vi "Top Level.vi"() -> ()   [LabVIEW 2020]
uses:
  Message.ctl
panel:
  in  "Reset DMM":bool
  out "Data":dbl
  in  "Close DMM":bool
  in  "Read DMM":bool
  in  "Init DMM":bool
  in  "Stop Button":bool
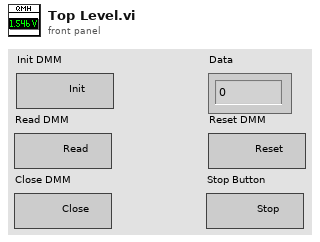
[diagram p1: front panel]
types:
  T1 = cluster{"NI":cluster{"Resource":refnum<k15>}, "Agilent":cluster{"Resource":refnum<visa-resource-name>}, "Data":dbl, "Data*":refnum<vi>, "DMM Type":string}
  T2 = typedef "Message.ctl" = cluster{"State":string, "Data":variant}
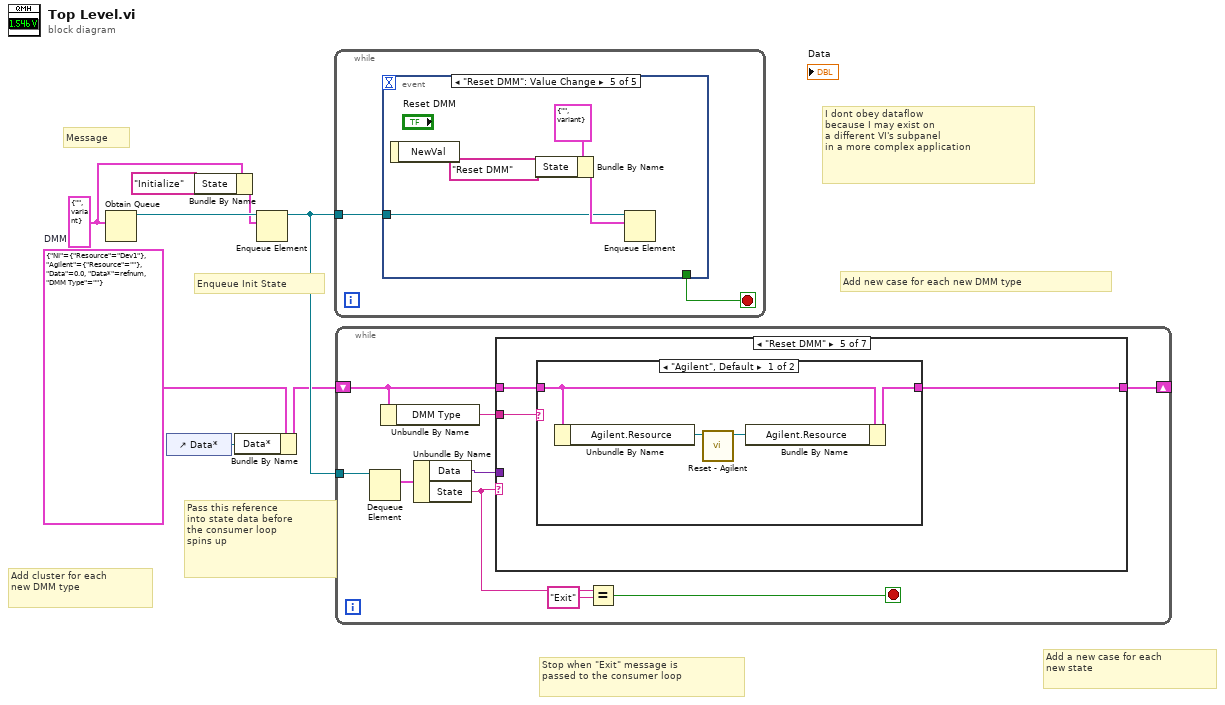
[diagram p0: block diagram]
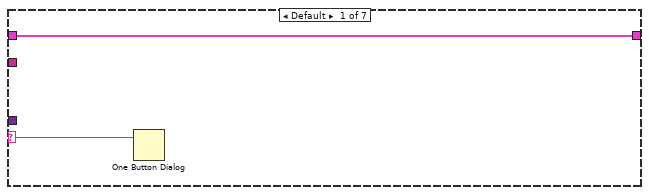
[diagram p2: hidden frame]
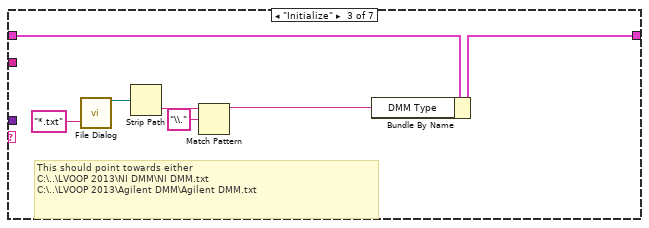
[diagram p4: hidden frame]
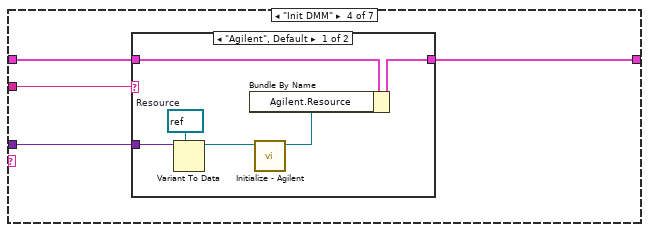
[diagram p5: hidden frame]
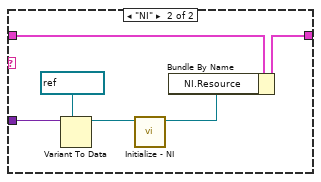
[diagram p6: hidden frame]
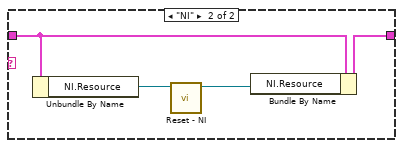
[diagram p7: hidden frame]
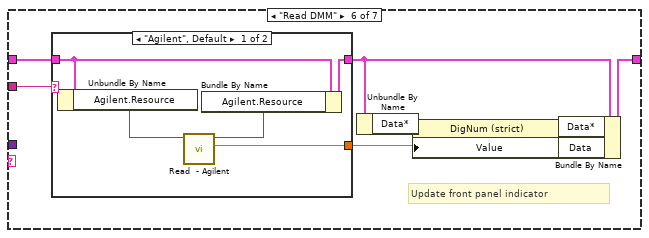
[diagram p8: hidden frame]
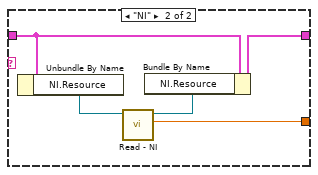
[diagram p9: hidden frame]
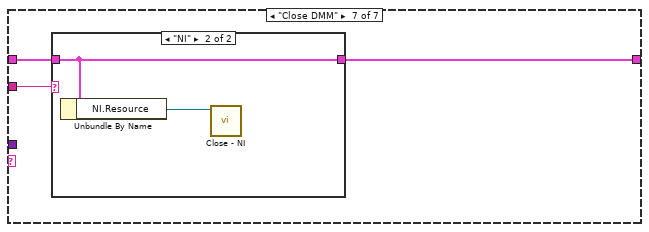
[diagram p10: hidden frame]
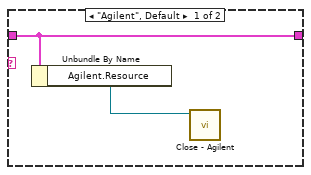
[diagram p11: hidden frame]
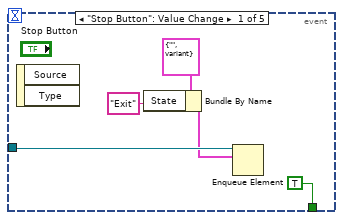
[diagram p12: hidden frame]
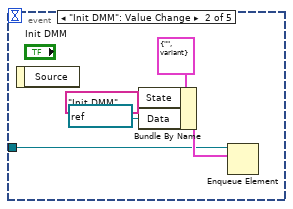
[diagram p13: hidden frame]
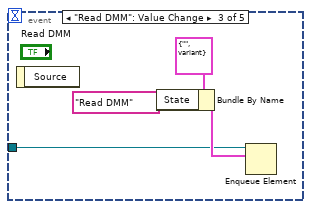
[diagram p14: hidden frame]
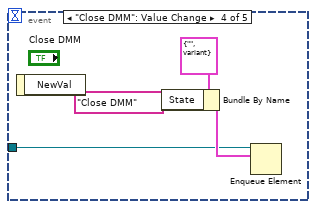
[diagram p15: hidden frame]
diagram:
  w3 = T1 {"NI"={"Resource"="Dev1"}, "Agilent"={"Resource"=""}, "Data"=0.0, "Data*"=refnum, "DMM Type"=""}  # DMM
  w6 = T2 {"State"="", "Data"=variant}
  # "I dont obey dataflow\nbecause I may exist on\na different VI's subpanel\nin a more complex application"
  # "Stop when \"Exit\" message is\npassed to the consumer loop"
  # "Add a new case for each\nnew state"
  # "Pass this reference\ninto state data before\nthe consumer loop\nspins up"
  # "Enqueue Init State"
  # "Add cluster for each\nnew DMM type"
  # "Add new case for each new DMM type"
  # "Message"
  n1 = Obtain Queue(element data type=w6) -> (queue out=w8:refnum<queue>)  [unwired: 4 in, 2 out]
  n2 = control-ref of="Data*"() -> (w1:refnum<vi>)
  n3 = Bundle By Name(cluster=w6, "State"="Initialize") -> (w5:T2)
  n4 = Bundle By Name(cluster=w3, "Data*"=w1) -> (w2:T1)
  n5 = Enqueue Element(queue=w8, element=w5) -> (queue out=w7:refnum<queue>)  [unwired: 2 in, 2 out]
  n6 = while {
    tunnel: w7 -> [w10]
    stop <- w9 stop-if-true
    n7 = event shown="[4] \"Reset DMM\": Value Change" {
      selector: _ -> [_ _ _ _ _]
      dyn-events: _ -> [_ _ _ _ _]
      timeout: _ -> [_ _ _ _ _]
      tunnel: w10 -> [w14 w17 w21 w25 w29]
      tunnel: [TRUE _ _ _ _] -> w9
      event "Stop Button": Value Change {
        n8 = event-data() -> ()  [unwired: 1 in, 2 out]
        n9 = Bundle By Name(cluster=T2 {"State"="", "Data"=variant}, "State"="Exit") -> (w12:T2)
        n10 = Enqueue Element(queue=w14, element=w12) -> ()  [unwired: 2 in, 3 out]
      }
      event "Init DMM": Value Change {
        n11 = event-data() -> ()  [unwired: 1 in, 1 out]
        n12 = Bundle By Name(cluster=T2 {"State"="", "Data"=variant}, "State"="Init DMM", "Data"=refnum<k15> "Dev1" ("Instrument Descriptor")) -> (w19:T2)
        n13 = Enqueue Element(queue=w17, element=w19) -> ()  [unwired: 2 in, 3 out]
      }
      event "Read DMM": Value Change {
        n14 = event-data() -> ()  [unwired: 1 in, 1 out]
        n15 = Bundle By Name(cluster=T2 {"State"="", "Data"=variant}, "State"="Read DMM") -> (w23:T2)
        n16 = Enqueue Element(queue=w21, element=w23) -> ()  [unwired: 2 in, 3 out]
      }
      event "Close DMM": Value Change {
        n17 = event-data() -> ()  [unwired: 1 in, 1 out]
        n18 = Bundle By Name(cluster=T2 {"State"="", "Data"=variant}, "State"="Close DMM") -> (w27:T2)
        n19 = Enqueue Element(queue=w25, element=w27) -> ()  [unwired: 2 in, 3 out]
      }
      event "Reset DMM": Value Change {
        n20 = event-data() -> ()  [unwired: 1 in, 1 out]
        n21 = Bundle By Name(cluster=T2 {"State"="", "Data"=variant}, "State"="Reset DMM") -> (w31:T2)
        n22 = Enqueue Element(queue=w29, element=w31) -> ()  [unwired: 2 in, 3 out]
      }
    }
  }
  n23 = while {
    tunnel: w7 -> [w41]
    shift-right: [w35] -> _
    shift-left: w2 -> [w34]
    stop <- w37 stop-if-true
    n24 = Dequeue Element(queue=w41) -> (element=w40:T2)  [unwired: 2 in, 3 out]
    n25 = Unbundle By Name(w34) -> ("DMM Type"=w33:string)
    n26 = Unbundle By Name(w40) -> ("Data"=w36:variant, "State"=w39:string)
    n27 = case shown="\"Reset DMM\"" w39 {
      selector: w39 -> [w43 _ _ _ _ _ _]
      tunnel: w36 -> [_ _ _ w53 _ _ _]
      tunnel: w34 -> [w42 w44 w51 w55 w70 w85 w98]
      tunnel: [w42 w44 w50 w54 w69 w83 w97] -> w35
      tunnel: w33 -> [_ _ _ w52 w68 w84 w96]
      frame Default {
        n28 = One Button Dialog(message=w43) -> ()  [unwired: 1 in, 1 out]
      }
      frame "Exit" {
      }
      frame "Initialize" {
        # "This should point towards either\nC:\\..\\LVOOP 2013\\NI DMM\\NI DMM.txt\nC:\\..\\LVOOP 2013\\Agilent DMM\\Agilent DMM.txt"
        n29 = call "File Dialog"("pattern (all files)"="*.txt") -> ("selected path"=w48:path)  [unwired: 11 in, 3 out]
        n30 = Strip Path(path=w48) -> (name=w47:string)  [unwired: 1 out]
        n31 = Match Pattern(string=w47, regular expression="\\.") -> (before substring=w45:string)  [unwired: 1 in, 3 out]
        n32 = Bundle By Name(cluster=w51, "DMM Type"=w45) -> (w50:T1)
      }
      frame "Init DMM" {
        n33 = case shown="\"Agilent\", Default" w52 {
          tunnel: w55 -> [w59 w65]
          tunnel: [w58 w64] -> w54
          tunnel: w53 -> [w60 w66]
          frame "Agilent", Default {
            w61 = refnum<visa-resource-name> refnum  # Resource
            n34 = Variant To Data(type=w61, Variant=w60) -> (data=w57:refnum<visa-resource-name>)  [unwired: 1 in, 1 out]
            n35 = call "Initialize - Agilent.vi"("VISA resource name"=w57) -> ("VISA resource name out"=w56:refnum<visa-resource-name>)  [unwired: 9 in, 1 out]
            n36 = Bundle By Name(cluster=w59, "Agilent.Resource"=w56) -> (w58:T1)
          }
          frame "NI" {
            n37 = Variant To Data(type=refnum<k15> "Dev1" ("Instrument Descriptor"), Variant=w66) -> (data=w63:refnum<k15>)  [unwired: 1 in, 1 out]
            n38 = call "Initialize - NI.vi"("Instrument Descriptor"=w63) -> ("instrument handle out"=w62:refnum<k15>)  [unwired: 9 in, 1 out]
            n39 = Bundle By Name(cluster=w65, "NI.Resource"=w62) -> (w64:T1)
          }
        }
      }
      frame "Reset DMM" {
        n40 = case shown="\"Agilent\", Default" w68 {
          tunnel: w70 -> [w73 w77]
          tunnel: [w74 w78] -> w69
          frame "Agilent", Default {
            n41 = Unbundle By Name(w73) -> ("Agilent.Resource"=w72:refnum<visa-resource-name>)
            n42 = call "Reset - Agilent.vi"("VISA resource name"=w72) -> ("VISA resource name out"=w71:refnum<visa-resource-name>)  [unwired: 9 in, 1 out]
            n43 = Bundle By Name(cluster=w73, "Agilent.Resource"=w71) -> (w74:T1)
          }
          frame "NI" {
            n44 = Unbundle By Name(w77) -> ("NI.Resource"=w76:refnum<k15>)
            n45 = call "Reset - NI.vi"("instrument handle"=w76) -> ("instrument handle out"=w75:refnum<k15>)  [unwired: 9 in, 1 out]
            n46 = Bundle By Name(cluster=w77, "NI.Resource"=w75) -> (w78:T1)
          }
        }
      }
      frame "Read DMM" {
        # "Update front panel indicator"
        n47 = case shown="\"Agilent\", Default" w84 {
          tunnel: w85 -> [w88 w94]
          tunnel: [w90 w95] -> w82
          tunnel: [w86 w91] -> w79
          frame "Agilent", Default {
            n48 = Unbundle By Name(w88) -> ("Agilent.Resource"=w87:refnum<visa-resource-name>)
            n49 = call "Read  - Agilent.vi"("VISA resource name"=w87) -> ("Measurement"=w86:dbl, "VISA resource name out"=w89:refnum<visa-resource-name>)  [unwired: 8 in, 1 out]
            n50 = Bundle By Name(cluster=w88, "Agilent.Resource"=w89) -> (w90:T1)
          }
          frame "NI" {
            n51 = Unbundle By Name(w94) -> ("NI.Resource"=w93:refnum<k15>)
            n52 = call "Read - NI.vi"("instrument handle"=w93) -> ("Measurement"=w91:dbl, "instrument handle out"=w92:refnum<k15>)  [unwired: 8 in, 1 out]
            n53 = Bundle By Name(cluster=w94, "NI.Resource"=w92) -> (w95:T1)
          }
        }
        n54 = Unbundle By Name(w82) -> ("Data*"=w81:refnum<vi>)
        n55 = property class="DigNum (strict)"(reference=w81, "Value"=w79) -> (reference out=w80:refnum<vi>)  [unwired: 1 in, 1 out]
        n56 = Bundle By Name(cluster=w82, "Data*"=w80, "Data"=w79) -> (w83:T1)
      }
      frame "Close DMM" {
        n57 = case shown="\"NI\"" w96 {
          tunnel: w98 -> [w100 w102]
          tunnel: [w100 w102] -> w97
          frame "Agilent", Default {
            n58 = Unbundle By Name(w100) -> ("Agilent.Resource"=w99:refnum<visa-resource-name>)
            n59 = call "Close - Agilent.vi"("VISA resource name"=w99) -> ()  [unwired: 10 in, 1 out]
          }
          frame "NI" {
            n60 = Unbundle By Name(w102) -> ("NI.Resource"=w101:refnum<k15>)
            n61 = call "Close - NI.vi"("instrument handle"=w101) -> ()  [unwired: 10 in, 1 out]
          }
        }
      }
    }
    n62 = Equal?(x=w39, y="Exit") -> (x = y?=w37:bool)
  }
